vi "Send Command SPI.vi"(0 "Tasks in":T1, 1 "rate":dbl, 2 "DUT1 Command/Write Frame":enum16{"Command Frame", "Data Frame"}(ring), 3 "DUT 1R/W":enum16{"Write", "Read"}(ring)=enum."Read", 4 "DUT 1Address":u16=2730 format="%.0x", 5 "error in (no error)":errorcluster, 6 "DUT 1Data":u16 format="%.0x") -> (14 "Tasks out":T1, 15 "Read value":u32, 19 "error out":errorcluster)   [LabVIEW 2023, in "SPI.lvlib"]
uses:
  SPI.lvlib
  Tasks.ctl
  1cdf4951-976b-4bd5-959a-79b185dea393.vi
  <vilib>/DAQmx/write.llb/DAQmx Write (Digital Bool 1Line 1Point).vi
  8bc3302b-2817-4b2c-89bb-4667548258a3.vi
  f01e5b01-51de-4428-ae73-5d681ac21d5e.vi
  <vilib>/DAQmx/write.llb/DAQmx Write (Digital Wfm 1Chan NSamp).vi
  <vilib>/DAQmx/read.llb/DAQmx Read (Digital Wfm 1Chan NSamp).vi
  <vilib>/Waveform/DWDTOps.llb/DWDT Boolean Array to Digital.vi
  <vilib>/DAQmx/miscellaneous.llb/DAQmx Fill In Error Info.vi
  <vilib>/Waveform/DWDTOps.llb/DWDT Uncompress Digital.vi
  <vilib>/Waveform/DWDTOps.llb/DWDT Digital to Boolean Array.vi
panel:
  out "DUT 1READ  array":bool[][](array[boolean])
  out "DUT1 WRITE":digitalwaveform(graph)={"t0"=timestamp(0 s since 1904-01-01), "dt"=0.0, "Y"={"transitions"=[], "data"=[]}, "error"={"status"=FALSE, "code"=37421928, "source"=""}}
  out "DUT 1READ":digitalwaveform(graph)={"t0"=timestamp(0 s since 1904-01-01), "dt"=0.0, "Y"={"transitions"=[], "data"=[]}, "error"={"status"=FALSE, "code"=37421928, "source"=""}}
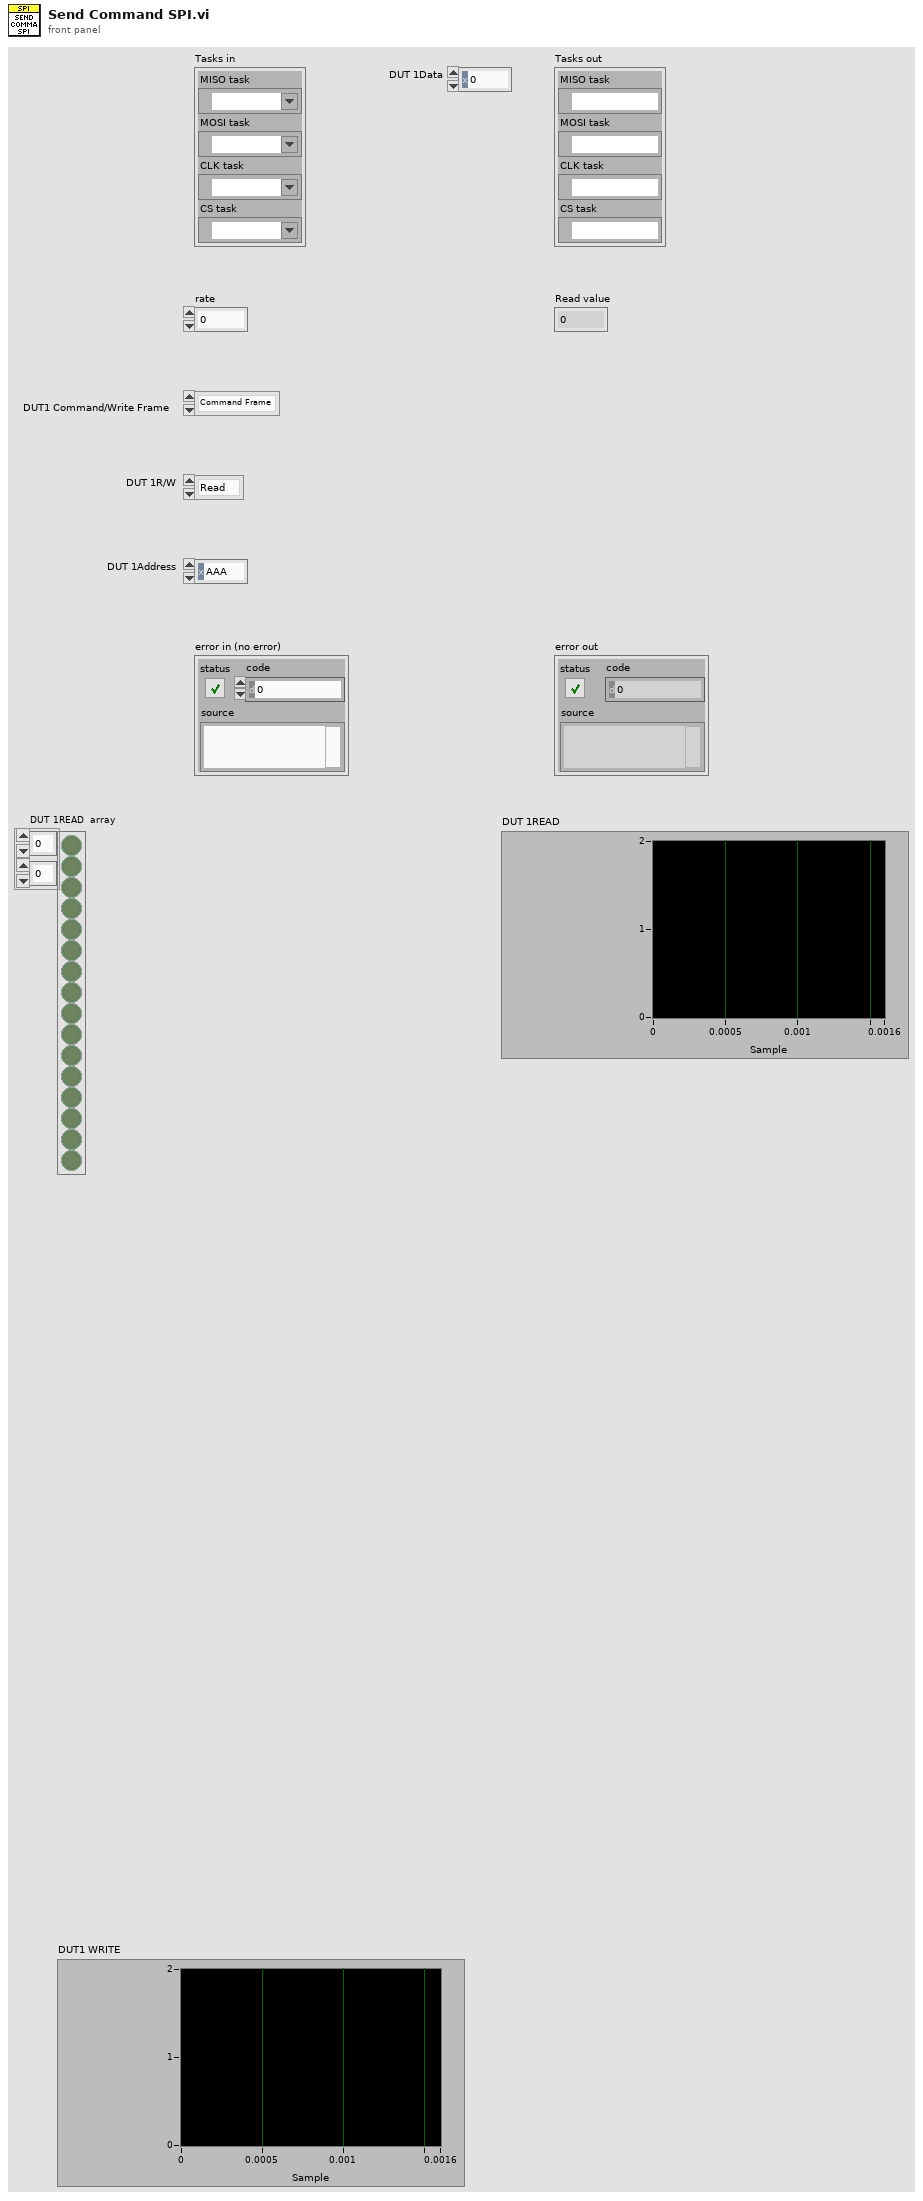
[diagram p1: front panel]
types:
  T1 = typedef "Tasks.ctl" = cluster{"MISO task":refnum<k21>, "MOSI task":refnum<k21>, "CLK task":refnum<k21>, "CS task":refnum<k21>}
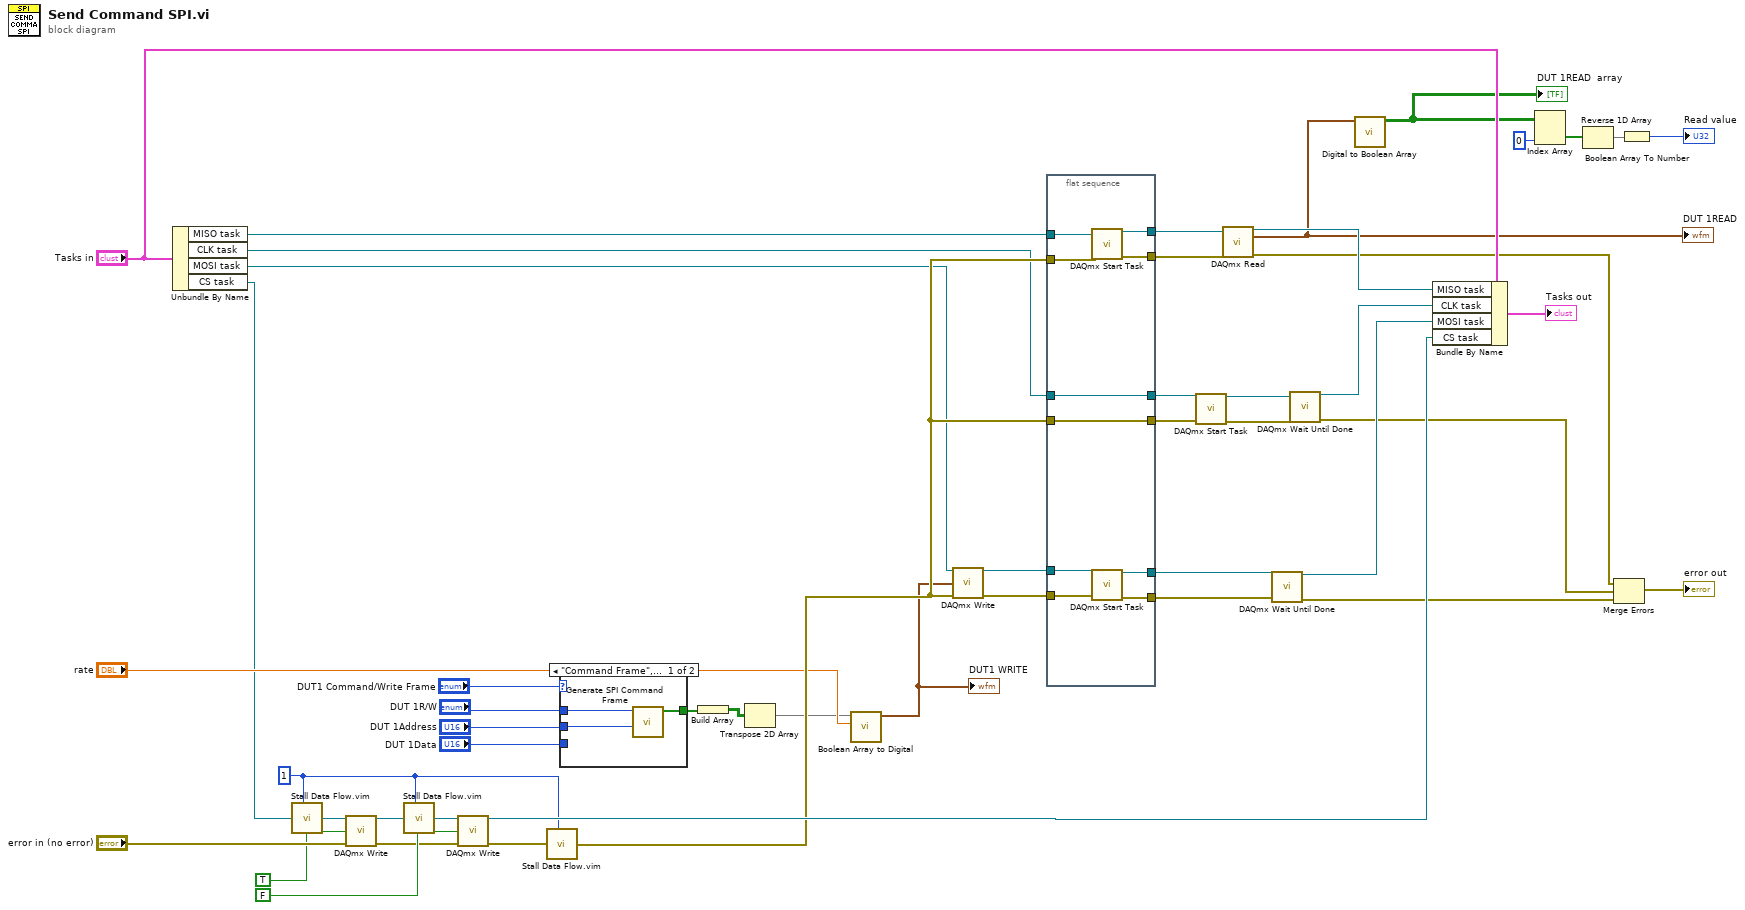
[diagram p0: block diagram]
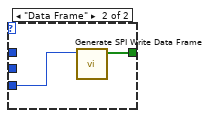
[diagram p2: hidden frame]
diagram:
  w33 = u32 1 ("milliseconds to wait")
  n1 = Unbundle By Name("Tasks in") -> ("MISO task"=w37:refnum<k21>, "CLK task"=w38:refnum<k21>, "MOSI task"=w39:refnum<k21>, "CS task"=w40:refnum<k21>)
  n2 = call "Stall Data Flow.vim"("value in"=w40, "milliseconds to wait"=w33) -> ("value out"=w27:refnum<k21>)  [unwired: 1 out]
  n3 = call-poly <vilib>:"DAQmx Write.vi"("task/channels in"=w27, "data"=TRUE, "error in"="error in (no error)") -> ("task out"=w28:refnum<k21>, "error out"=w30:errorcluster)  [unwired: 10 in, 1 out]
  n4 = call "Stall Data Flow.vim"("value in"=w28, "milliseconds to wait"=w33) -> ("value out"=w29:refnum<k21>)  [unwired: 1 out]
  n5 = call-poly <vilib>:"DAQmx Write.vi"("task/channels in"=w29, "data"=FALSE, "error in"=w30) -> ("task out"=w49:refnum<k21>, "error out"=w31:errorcluster)  [unwired: 10 in, 1 out]
  n6 = call "Stall Data Flow.vim"("value in"=w31, "milliseconds to wait"=w33) -> ("value out"=w43:errorcluster)  [unwired: 1 out]
  n7 = case shown="\"Command Frame\", Default" "DUT1 Command/Write Frame" {
    tunnel: "DUT 1R/W" -> [w52 _]
    tunnel: "DUT 1Address" -> [w51 _]
    tunnel: [w50 w53] -> w19
    tunnel: "DUT 1Data" -> [_ w54]
    frame "Command Frame", Default {
      n8 = call "Generate SPI Command Frame.vi"("Address"=w51, "R/W"=w52) -> ("SPI Command Frame"=w50:bool[])  [unwired: 9 in]
    }
    frame "Data Frame" {
      n9 = call "Generate SPI Write Data Frame.vi"("Data"=w54) -> ("SPI Write Data Frame"=w53:bool[])  [unwired: 10 in]
    }
  }
  n10 = Build Array(w19) -> (w20:bool[][])
  n11 = Transpose 2D Array(2D array=w20) -> (transposed array=w21:bool[][])
  n12 = call-poly <vilib>:"Boolean Array to Digital.vi"("sample rate"="rate", "boolean array"=w21) -> ("digital waveform"=w8:digitalwaveform)  [unwired: 8 in, 1 out]
  "DUT1 WRITE" <- w8
  n13 = call-poly <vilib>:"DAQmx Write.vi"("task/channels in"=w39, "data"=w8, "error in"=w43) -> ("task out"=w7:refnum<k21>, "error out"=w11:errorcluster)  [unwired: 10 in, 1 out]
  n14 = flat-sequence {
    tunnel: w37 -> [w64]
    tunnel: w43 -> [w63]
    tunnel: [w62] -> w5
    tunnel: [w61] -> w6
    tunnel: w7 -> [w60]
    tunnel: [w59] -> w9
    tunnel: [w58] -> w10
    tunnel: w11 -> [w57]
    tunnel: w38 -> [w56]
    tunnel: w43 -> [w55]
    tunnel: [w56] -> w12
    tunnel: [w55] -> w13
    frame #0 {
      n15 = call <vilib>:"DAQmx Start Task.vi"("task/channels in"=w64, "error in"=w63) -> ("task out"=w61:refnum<k21>, "error out"=w59:errorcluster)  [unwired: 12 in]
      n16 = call <vilib>:"DAQmx Start Task.vi"("task/channels in"=w60, "error in"=w57) -> ("task out"=w62:refnum<k21>, "error out"=w58:errorcluster)  [unwired: 12 in]
    }
  }
  n17 = call <vilib>:"DAQmx Start Task.vi"("task/channels in"=w12, "error in"=w13) -> ("task out"=w14:refnum<k21>, "error out"=w15:errorcluster)  [unwired: 12 in]
  n18 = call-poly <vilib>:"DAQmx Read.vi"("task/channels in"=w6, "error in"=w9) -> ("task out"=w46:refnum<k21>, "data"=w16:digitalwaveform, "error out"=w4:errorcluster)  [unwired: 11 in]
  "DUT 1READ" <- w16
  n19 = call <vilib>:"DAQmx Wait Until Done.vi"("task/channels in"=w5, "error in"=w10) -> ("task out"=w48:refnum<k21>, "error out"=w1:errorcluster)  [unwired: 12 in]
  n20 = call <vilib>:"DAQmx Wait Until Done.vi"("task/channels in"=w14, "error in"=w15) -> ("task out"=w47:refnum<k21>, "error out"=w3:errorcluster)  [unwired: 12 in]
  n21 = call-poly <vilib>:"Digital to Boolean Array.vi"("digital waveform"=w16) -> ("boolean array"=w22:bool[][])  [unwired: 9 in, 1 out]
  "DUT 1READ  array" <- w22
  n22 = Bundle By Name(cluster="Tasks in", "MISO task"=w46, "CLK task"=w47, "MOSI task"=w48, "CS task"=w49) -> (→"Tasks out":T1)
  n23 = Index Array(array=w22, index (col)=0 ("disabled index (col)")) -> (element=w25:bool[])  [unwired: 1 in]
  n24 = Reverse 1D Array(array=w25) -> (reversed array=w26:bool[])
  n25 = Merge Errors(w4, w3, w1) -> (→"error out":errorcluster)
  n26 = Boolean Array To Number(Boolean array=w26) -> (number=→"Read value":u32)
